vi "GetType.vi"(8 "error in (no error)":errorcluster, 11 "Configure Output Impedance Msg":refnum<class "Configure Output Impedance Msg.lvclass">) -> (0 "error out":errorcluster, 2 "Data Sample":variant, 3 "Configure Output Impedance Msg":refnum<class "Configure Output Impedance Msg.lvclass">)   [LabVIEW 2016, in "CS++Fgen.lvlib" / "Configure Output Impedance Msg.lvclass"]
doc: "This VI delivers a sample of the data type format the message expects."
uses:
  Configure Output Impedance Msg.lvclass
  Configure Output Impedance Msg.lvclass/Configure Output Impedance Msg.ctl
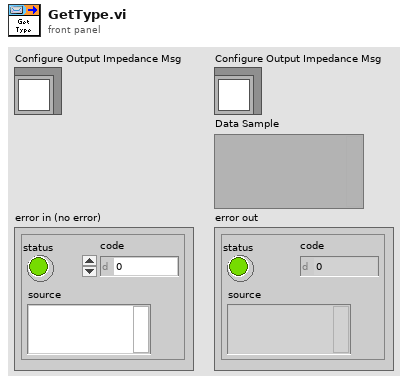
[diagram p1: front panel]
types:
  T1 = cluster{"channel name (\"CHANNEL1\")":string, "impedance (50 Ohms)":dbl[unit]}
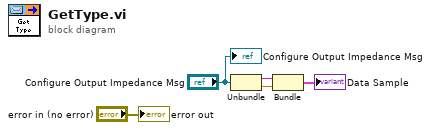
[diagram p0: block diagram]
diagram:
  n1 = Unbundle("Configure Output Impedance Msg") -> (w2:string, w1:dbl[unit])
  n2 = Bundle("channel name (\"CHANNEL1\")"=w2, "impedance (50 Ohms)"=w1) -> (→"Data Sample":T1)  [unwired: 1 in]
  "error out" <- "error in (no error)"
  "Configure Output Impedance Msg" <- "Configure Output Impedance Msg"
